vi "rad_PackageImage.vi"(7 "AppImage Properties.FPGA Properties":T1, 8 "error in (no error)":errorcluster, 9 "AppImage Path":path, 10 "Temp Image Path":path, 11 "App Image Info File Path":path) -> (0 "error out":errorcluster)   [LabVIEW 2014]
uses:
  TypeDefs/rad_FPGA Properties.ctl
  TypeDefs/rad_FPGA Flash Properties.ctl
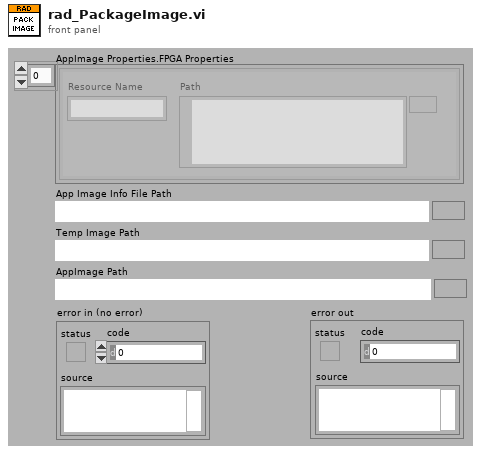
[diagram p1: front panel]
types:
  T1 = typedef "rad_FPGA Properties.ctl" = T2[]
  T2 = typedef "rad_FPGA Flash Properties.ctl" = cluster{"Resource Name":string, "Path":path}
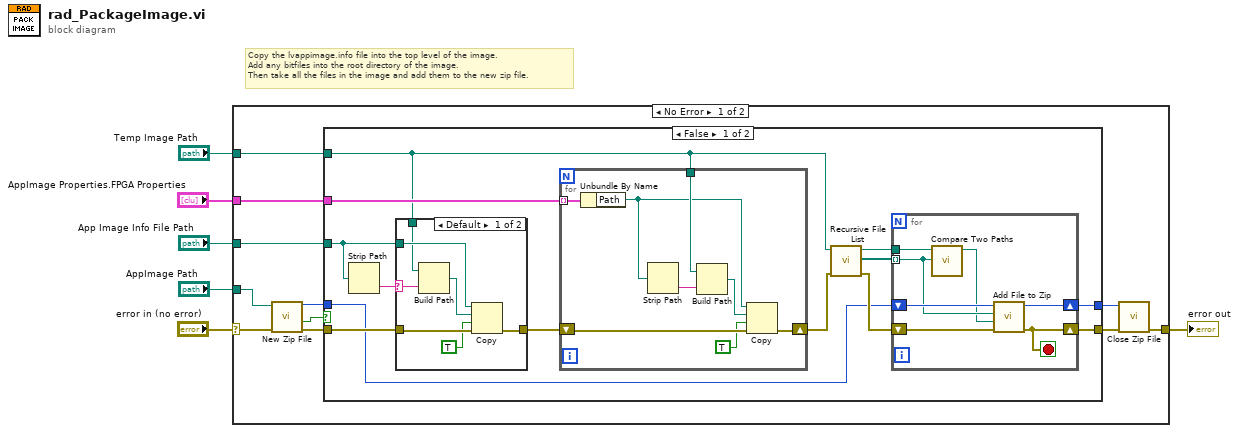
[diagram p0: block diagram]
diagram:
  # "Copy the lvappimage.info file into the top level of the image.\nAdd any bitfiles into the root directory of the image.\nThen take all the files in the image and add them to the new zip file."
  n1 = case shown="No Error" "error in (no error)" {
    selector: "error in (no error)" -> [w8 w56]
    tunnel: "App Image Info File Path" -> [w14 _]
    tunnel: "AppImage Properties.FPGA Properties" -> [w13 _]
    tunnel: "Temp Image Path" -> [w12 _]
    tunnel: [w9 w56] -> w2
    tunnel: "AppImage Path" -> [w7 _]
    frame No Error {
      n2 = call <vilib>:"New Zip File.vi"("error in (no error)"=w8, "target"=w7) -> ("error out"=w16:errorcluster, "cancelled"=w15:bool, "zip file out"=w17:i64)  [unwired: 3 in]
      n3 = case shown="False" w15 {
        tunnel: w17 -> [w18 w54]
        tunnel: w16 -> [w26 w55]
        tunnel: [w21 w55] -> w10
        tunnel: [w20 w54] -> w11
        tunnel: w14 -> [w29 _]
        tunnel: w13 -> [w28 _]
        tunnel: w12 -> [w19 _]
        frame False {
          n4 = Strip Path(path=w29) -> (name=w27:string)  [unwired: 1 out]
          n5 = case shown="Default" w27 {
            selector: w27 -> [w41 _]
            tunnel: w26 -> [w43 w45]
            tunnel: [w44 w45] -> w30
            tunnel: w29 -> [w42 _]
            tunnel: w19 -> [w40 _]
            frame Default {
              n6 = Build Path(base path=w40, name or relative path=w41) -> (appended path=w39:path)
              n7 = Copy(8:w43, 9:TRUE ("overwrite (F)"), 10:w39, 11:w42) -> (0:w44:errorcluster)  [unwired: 1 in, 2 out]
            }
            frame "" {
            }
          }
          n8 = for {
            tunnel: w28 -> [w53] mode=indexing
            shift-right: [w52] -> w25
            shift-left: w30 -> [w51]
            tunnel: w19 -> [w49]
            n9 = Unbundle By Name(w53) -> ("Path"=w48:path)
            n10 = Strip Path(path=w48) -> (name=w50:string)  [unwired: 1 out]
            n11 = Build Path(base path=w49, name or relative path=w50) -> (appended path=w47:path)
            n12 = Copy(8:w51, 9:TRUE ("overwrite (F)"), 10:w47, 11:w48) -> (0:w52:errorcluster)  [unwired: 1 in, 2 out]
          }
          n13 = call <vilib>:"Recursive File List.vi"("error in (no error)"=w25, "Folder Path"=w19) -> ("error out"=w24:errorcluster, "All Files in Dir"=w22:path[], "dup Folder Path"=w23:path)  [unwired: 1 in, 6 out]
          n14 = for {
            tunnel: w22 -> [w33] mode=indexing
            shift-right: [w35] -> w20
            shift-left: w18 -> [w37]
            shift-right: [w34] -> w21
            shift-left: w24 -> [w36]
            tunnel: w23 -> [w31]
            stop <- w34 stop-if-true
            n15 = call <vilib>:"Compare Two Paths.vi"("Path 2"=w33, "Path 1"=w31) -> ("Relative Path from 1 to 2"=w32:path)  [unwired: 1 in, 8 out]
            n16 = call <vilib>:"Add File to Zip.vi"("error in (no error)"=w36, "destination path in zip"=w32, "source file path"=w33, "zip file in"=w37) -> ("error out"=w34:errorcluster, "zip file out"=w35:i64)  [unwired: 6 out]
          }
        }
        frame True {
        }
      }
      n17 = call <vilib>:"Close Zip File.vi"("error in (no error)"=w10, "zip file in"=w11) -> ("error out"=w9:errorcluster)  [unwired: 5 in]
    }
    frame Error {
    }
  }
  "error out" <- w2
